vi "Chroma 1905x Series Get Preset Configuration.vi"(0 "inst handle in":refnum<visa-resource-name>, 5 "error in":T1) -> (6 "Pass Judgement Time":string, 7 "GFI":string, 8 "Step Wait Time":string, 9 "Part Number":string, 10 "Time before Judgement":string, 11 "Lot Number":string, 12 "Offset":string, 13 "Serial Number":string, 14 "inst handle out":refnum<visa-resource-name>, 15 "Low Limit":string, 16 "AutoRanging":string, 17 "Automatic Gain Control":string, 18 "Ground Continuity":string, 19 "error out":T1)   [LabVIEW 2025]
doc: "Contact Chroma\nTEL: +886-2-2298-3855 \nTEL: +886-3-397-5788 \nFAX: +886-2-2298-3596\nFAX: +886-3-327-4703 \nURL: http://www.chromaate.com \nE-mail: chroma@chroma.com.tw"
uses:
  <instrlib>/Chroma 19052/Chroma 19052.lvlib
panel:
  # "Get Configuration Screen"
  # "Get Preset Configuration"
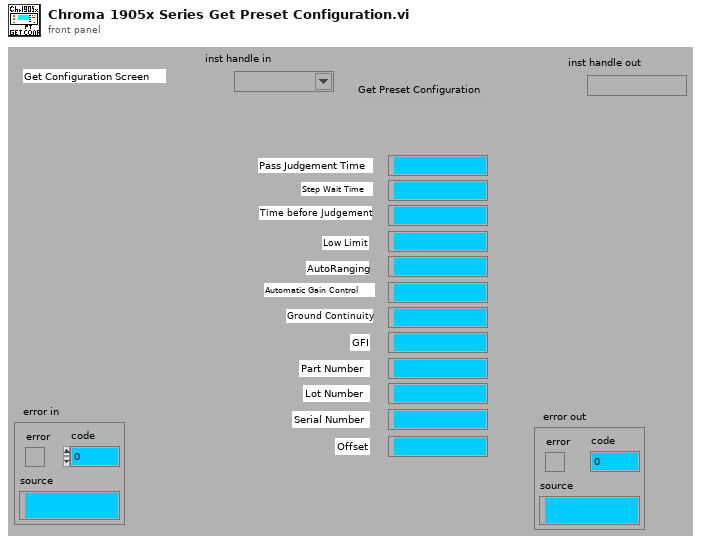
[diagram p1: front panel]
types:
  T1 = cluster{"error":bool, "code":i8, "source":string}
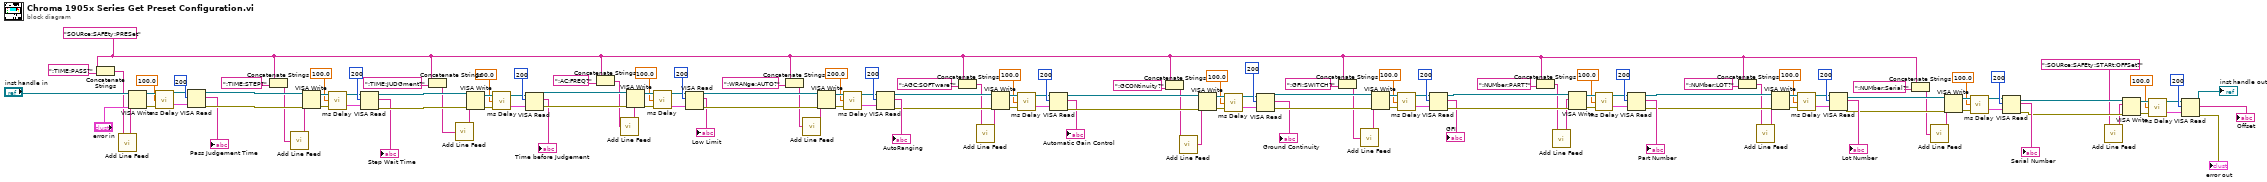
[diagram p0: block diagram]
diagram:
  w29 = "SOURce:SAFEty:PRESet" ("string (\"\")")
  n1 = Concatenate Strings(w29, ":TIME:PASS?") -> (w22:string)
  n2 = call <instrlib>:"Add Line Feed.vi"("Cmdstring"=w22) -> ("Concatenated String"=w21:string)
  n3 = VISA Write(VISA resource name="inst handle in", write buffer=w21, error in (no error)="error in") -> (VISA resource name out=w140:refnum<visa-resource-name>, error out=w143:errorcluster)  [unwired: 1 out]
  n4 = call <instrlib>:"ms Delay.vi"("error in"=w143, "Time Delay S"=100.0, "inst handle in"=w140) -> ("error out"=w142:T1, "inst handle Out"=w141:refnum<visa-resource-name>)
  n5 = VISA Read(VISA resource name=w141, byte count=u32 200 ("byte count (0)"), error in (no error)=w142) -> (VISA resource name out=w131:refnum<visa-resource-name>, read buffer=→"Pass Judgement Time":string, error out=w130:errorcluster)  [unwired: 1 out]
  n6 = Concatenate Strings(w29, ":TIME:STEP?") -> (w20:string)
  n7 = call <instrlib>:"Add Line Feed.vi"("Cmdstring"=w20) -> ("Concatenated String"=w19:string)
  n8 = VISA Write(VISA resource name=w131, write buffer=w19, error in (no error)=w130) -> (VISA resource name out=w133:refnum<visa-resource-name>, error out=w136:errorcluster)  [unwired: 1 out]
  n9 = call <instrlib>:"ms Delay.vi"("error in"=w136, "Time Delay S"=100.0, "inst handle in"=w133) -> ("error out"=w135:T1, "inst handle Out"=w134:refnum<visa-resource-name>)
  n10 = VISA Read(VISA resource name=w134, byte count=u32 200 ("byte count (0)"), error in (no error)=w135) -> (VISA resource name out=w122:refnum<visa-resource-name>, read buffer=→"Step Wait Time":string, error out=w123:errorcluster)  [unwired: 1 out]
  n11 = Concatenate Strings(w29, ":TIME:JUDGment?") -> (w18:string)
  n12 = call <instrlib>:"Add Line Feed.vi"("Cmdstring"=w18) -> ("Concatenated String"=w17:string)
  n13 = VISA Write(VISA resource name=w122, write buffer=w17, error in (no error)=w123) -> (VISA resource name out=w125:refnum<visa-resource-name>, error out=w128:errorcluster)  [unwired: 1 out]
  n14 = call <instrlib>:"ms Delay.vi"("error in"=w128, "Time Delay S"=100.0, "inst handle in"=w125) -> ("error out"=w127:T1, "inst handle Out"=w126:refnum<visa-resource-name>)
  n15 = VISA Read(VISA resource name=w126, byte count=u32 200 ("byte count (0)"), error in (no error)=w127) -> (VISA resource name out=w113:refnum<visa-resource-name>, read buffer=→"Time before Judgement":string, error out=w114:errorcluster)  [unwired: 1 out]
  n16 = Concatenate Strings(w29, ":AC:FREQ?") -> (w16:string)
  n17 = call <instrlib>:"Add Line Feed.vi"("Cmdstring"=w16) -> ("Concatenated String"=w15:string)
  n18 = VISA Write(VISA resource name=w113, write buffer=w15, error in (no error)=w114) -> (VISA resource name out=w116:refnum<visa-resource-name>, error out=w119:errorcluster)  [unwired: 1 out]
  n19 = call <instrlib>:"ms Delay.vi"("error in"=w119, "Time Delay S"=100.0, "inst handle in"=w116) -> ("error out"=w118:T1, "inst handle Out"=w117:refnum<visa-resource-name>)
  n20 = VISA Read(VISA resource name=w117, byte count=u32 200 ("byte count (0)"), error in (no error)=w118) -> (VISA resource name out=w104:refnum<visa-resource-name>, read buffer=→"Low Limit":string, error out=w105:errorcluster)  [unwired: 1 out]
  n21 = Concatenate Strings(w29, ":WRANge:AUTO?") -> (w14:string)
  n22 = call <instrlib>:"Add Line Feed.vi"("Cmdstring"=w14) -> ("Concatenated String"=w13:string)
  n23 = VISA Write(VISA resource name=w104, write buffer=w13, error in (no error)=w105) -> (VISA resource name out=w107:refnum<visa-resource-name>, error out=w110:errorcluster)  [unwired: 1 out]
  n24 = call <instrlib>:"ms Delay.vi"("error in"=w110, "Time Delay S"=200.0, "inst handle in"=w107) -> ("error out"=w109:T1, "inst handle Out"=w108:refnum<visa-resource-name>)
  n25 = VISA Read(VISA resource name=w108, byte count=u32 200 ("byte count (0)"), error in (no error)=w109) -> (VISA resource name out=w68:refnum<visa-resource-name>, read buffer=→"AutoRanging":string, error out=w64:errorcluster)  [unwired: 1 out]
  n26 = Concatenate Strings(w29, ":AGC:SOFTware?") -> (w12:string)
  n27 = call <instrlib>:"Add Line Feed.vi"("Cmdstring"=w12) -> ("Concatenated String"=w11:string)
  n28 = VISA Write(VISA resource name=w68, write buffer=w11, error in (no error)=w64) -> (VISA resource name out=w94:refnum<visa-resource-name>, error out=w97:errorcluster)  [unwired: 1 out]
  n29 = call <instrlib>:"ms Delay.vi"("error in"=w97, "Time Delay S"=100.0, "inst handle in"=w94) -> ("error out"=w96:T1, "inst handle Out"=w95:refnum<visa-resource-name>)
  n30 = VISA Read(VISA resource name=w95, byte count=u32 200 ("byte count (0)"), error in (no error)=w96) -> (VISA resource name out=w69:refnum<visa-resource-name>, read buffer=→"Automatic Gain Control":string, error out=w67:errorcluster)  [unwired: 1 out]
  n31 = Concatenate Strings(w29, ":GCONtinuity?") -> (w10:string)
  n32 = call <instrlib>:"Add Line Feed.vi"("Cmdstring"=w10) -> ("Concatenated String"=w9:string)
  n33 = VISA Write(VISA resource name=w69, write buffer=w9, error in (no error)=w67) -> (VISA resource name out=w87:refnum<visa-resource-name>, error out=w90:errorcluster)  [unwired: 1 out]
  n34 = call <instrlib>:"ms Delay.vi"("error in"=w90, "Time Delay S"=100.0, "inst handle in"=w87) -> ("error out"=w89:T1, "inst handle Out"=w88:refnum<visa-resource-name>)
  n35 = VISA Read(VISA resource name=w88, byte count=u32 200 ("byte count (0)"), error in (no error)=w89) -> (VISA resource name out=w70:refnum<visa-resource-name>, read buffer=→"Ground Continuity":string, error out=w65:errorcluster)  [unwired: 1 out]
  n36 = Concatenate Strings(w29, ":GFI:SWITCH?") -> (w8:string)
  n37 = call <instrlib>:"Add Line Feed.vi"("Cmdstring"=w8) -> ("Concatenated String"=w7:string)
  n38 = VISA Write(VISA resource name=w70, write buffer=w7, error in (no error)=w65) -> (VISA resource name out=w80:refnum<visa-resource-name>, error out=w83:errorcluster)  [unwired: 1 out]
  n39 = call <instrlib>:"ms Delay.vi"("error in"=w83, "Time Delay S"=100.0, "inst handle in"=w80) -> ("error out"=w82:T1, "inst handle Out"=w81:refnum<visa-resource-name>)
  n40 = VISA Read(VISA resource name=w81, byte count=u32 200 ("byte count (0)"), error in (no error)=w82) -> (VISA resource name out=w71:refnum<visa-resource-name>, read buffer=→"GFI":string, error out=w66:errorcluster)  [unwired: 1 out]
  n41 = Concatenate Strings(w29, ":NUMber:PART?") -> (w6:string)
  n42 = call <instrlib>:"Add Line Feed.vi"("Cmdstring"=w6) -> ("Concatenated String"=w5:string)
  n43 = VISA Write(VISA resource name=w71, write buffer=w5, error in (no error)=w66) -> (VISA resource name out=w73:refnum<visa-resource-name>, error out=w76:errorcluster)  [unwired: 1 out]
  n44 = call <instrlib>:"ms Delay.vi"("error in"=w76, "Time Delay S"=100.0, "inst handle in"=w73) -> ("error out"=w75:T1, "inst handle Out"=w74:refnum<visa-resource-name>)
  n45 = VISA Read(VISA resource name=w74, byte count=u32 200 ("byte count (0)"), error in (no error)=w75) -> (VISA resource name out=w39:refnum<visa-resource-name>, read buffer=→"Part Number":string, error out=w38:errorcluster)  [unwired: 1 out]
  n46 = Concatenate Strings(w29, ":NUMber:LOT?") -> (w4:string)
  n47 = call <instrlib>:"Add Line Feed.vi"("Cmdstring"=w4) -> ("Concatenated String"=w3:string)
  n48 = VISA Write(VISA resource name=w39, write buffer=w3, error in (no error)=w38) -> (VISA resource name out=w52:refnum<visa-resource-name>, error out=w55:errorcluster)  [unwired: 1 out]
  n49 = call <instrlib>:"ms Delay.vi"("error in"=w55, "Time Delay S"=100.0, "inst handle in"=w52) -> ("error out"=w54:T1, "inst handle Out"=w53:refnum<visa-resource-name>)
  n50 = VISA Read(VISA resource name=w53, byte count=u32 200 ("byte count (0)"), error in (no error)=w54) -> (VISA resource name out=w41:refnum<visa-resource-name>, read buffer=→"Lot Number":string, error out=w40:errorcluster)  [unwired: 1 out]
  n51 = Concatenate Strings(w29, ":NUMber:Serial?") -> (w2:string)
  n52 = call <instrlib>:"Add Line Feed.vi"("Cmdstring"=w2) -> ("Concatenated String"=w1:string)
  n53 = VISA Write(VISA resource name=w41, write buffer=w1, error in (no error)=w40) -> (VISA resource name out=w44:refnum<visa-resource-name>, error out=w47:errorcluster)  [unwired: 1 out]
  n54 = call <instrlib>:"ms Delay.vi"("error in"=w47, "Time Delay S"=100.0, "inst handle in"=w44) -> ("error out"=w46:T1, "inst handle Out"=w45:refnum<visa-resource-name>)
  n55 = VISA Read(VISA resource name=w45, byte count=u32 200 ("byte count (0)"), error in (no error)=w46) -> (VISA resource name out=w30:refnum<visa-resource-name>, read buffer=→"Serial Number":string, error out=w31:errorcluster)  [unwired: 1 out]
  n56 = call <instrlib>:"Add Line Feed.vi"("Cmdstring"=":SOURce:SAFEty:STARt:OFFSet?") -> ("Concatenated String"=w24:string)
  n57 = VISA Write(VISA resource name=w30, write buffer=w24, error in (no error)=w31) -> (VISA resource name out=w33:refnum<visa-resource-name>, error out=w36:errorcluster)  [unwired: 1 out]
  n58 = call <instrlib>:"ms Delay.vi"("error in"=w36, "Time Delay S"=100.0, "inst handle in"=w33) -> ("error out"=w35:T1, "inst handle Out"=w34:refnum<visa-resource-name>)
  n59 = VISA Read(VISA resource name=w34, byte count=u32 200 ("byte count (0)"), error in (no error)=w35) -> (VISA resource name out=→"inst handle out":refnum<visa-resource-name>, read buffer=→"Offset":string, error out=→"error out":errorcluster)  [unwired: 1 out]
